vi "Máscaras registros.vi"(7 "Espera acceso USB:":u32, 8 "error in":errorcluster, 9 "Sumador-Salida":i32, 10 "Canal":i32, 11 "ftHandle_in":u32) -> (0 "error out":errorcluster, 1 "Scaler":i32, 2 "Num registro":i32, 3 "ftHandle_out":u32, 4 "DAC_MUX ENA":u16)   [LabVIEW 2009]
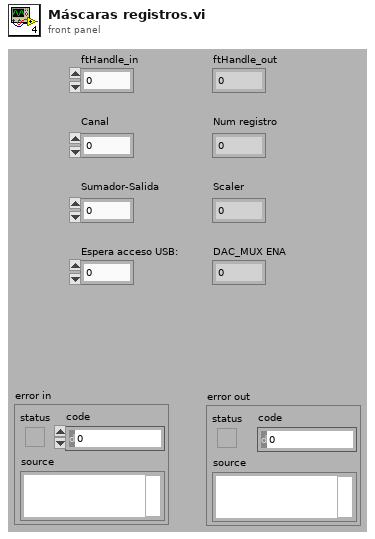
[diagram p1: front panel]
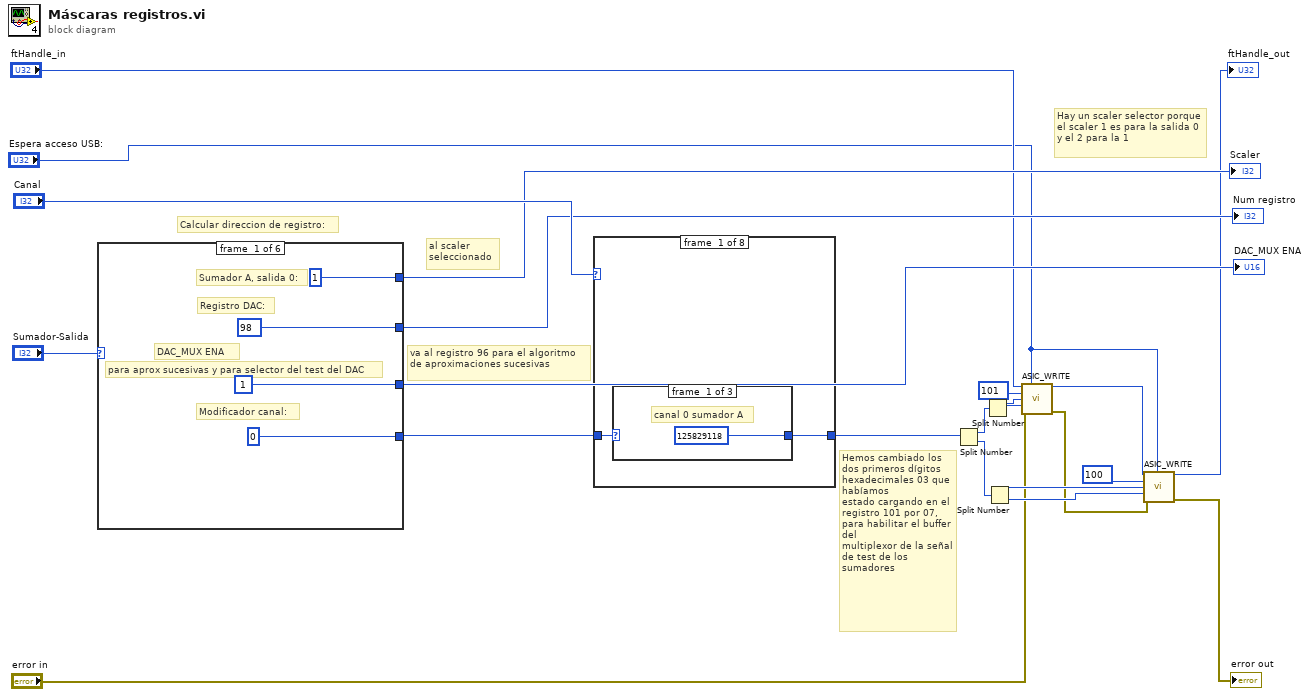
[diagram p0: block diagram]
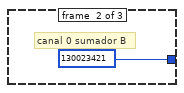
[diagram p2: hidden frame]
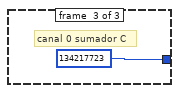
[diagram p3: hidden frame]
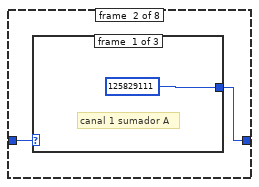
[diagram p4: hidden frame]
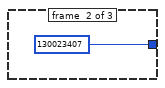
[diagram p5: hidden frame]
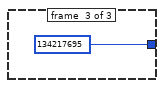
[diagram p6: hidden frame]
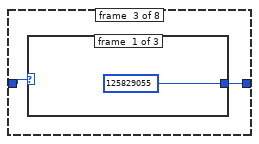
[diagram p7: hidden frame]
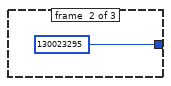
[diagram p8: hidden frame]
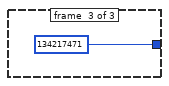
[diagram p9: hidden frame]
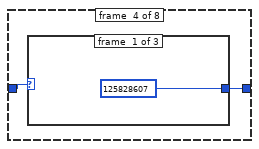
[diagram p10: hidden frame]
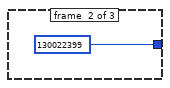
[diagram p11: hidden frame]
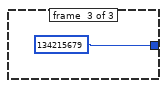
[diagram p12: hidden frame]
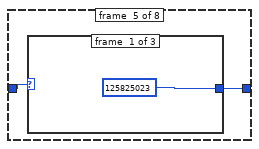
[diagram p13: hidden frame]
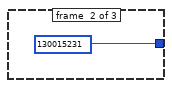
[diagram p14: hidden frame]
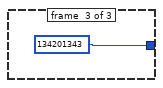
[diagram p15: hidden frame]
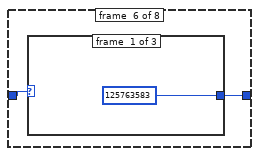
[diagram p16: hidden frame]
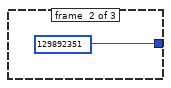
[diagram p17: hidden frame]
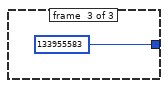
[diagram p18: hidden frame]
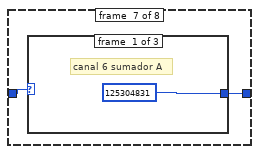
[diagram p19: hidden frame]
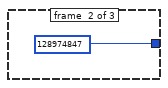
[diagram p20: hidden frame]
diagram:
  # "Hemos cambiado los dos primeros dígitos hexadecimales 03 que habíamos\nestado cargando en el registro 101 por 07, para habilitar el buffer del \nmultiplexor de la señal de test de los sumadores"
  # "Hay un scaler selector porque el scaler 1 es para la salida 0 y el 2 para la 1"
  # "al scaler\nseleccionado"
  # "va al registro 96 para el algoritmo de aproximaciones sucesivas"
  # "Calcular direccion de registro:"
  n1 = case shown="0, Default" "Sumador-Salida" {
    tunnel: [98 99 97 98 99 97] -> w12
    tunnel: [u16 1 2 3 4 5 6] -> w10
    tunnel: [0 1 2 0 1 2] -> w14
    tunnel: [1 1 1 2 2 2] -> w11
    frame #0 {
      # "para aprox sucesivas y para selector del test del DAC"
      # "Modificador canal:"
      # "DAC_MUX ENA"
      # "Registro DAC:"
      # "Sumador A, salida 0:"
    }
    frame #1 {
      # "Modificador canal:"
      # "Registro DAC:"
      # "Sumador B, salida 0:"
    }
    frame #2 {
      # "Modificador canal:"
      # "Registro DAC:"
      # "Sumador C, salida 0:"
    }
    frame #3 {
      # "Modificador canal:"
      # "Registro DAC:"
      # "Sumador A, salida 1:"
    }
    frame #4 {
      # "Modificador canal:"
      # "Registro DAC:"
      # "Sumador B, salida 1:"
    }
    frame #5 {
      # "Modificador canal:"
      # "Registro DAC:"
      # "Sumador C, salida 1:"
    }
  }
  "Num registro" <- w12
  "Scaler" <- w11
  "DAC_MUX ENA" <- w10
  n2 = case shown="1" "Canal" {
    tunnel: w14 -> [w48 w53 w58 w63 w68 w73 w78 w83]
    tunnel: [w47 w52 w57 w62 w67 w72 w77 w82] -> w1
    frame #0 {
      n3 = case shown="0, Default" w48 {
        tunnel: [u32 125829118 ("Threshold Inicial N") u32 130023421 ("Threshold Inicial N") u32 134217723 ("Threshold Inicial N")] -> w47
        frame #0 {
          # "canal 0 sumador A"
        }
        frame #1 {
          # "canal 0 sumador B"
        }
        frame #2 {
          # "canal 0 sumador C"
        }
      }
    }
    frame #1 {
      n4 = case shown="0, Default" w53 {
        tunnel: [u32 125829111 ("Threshold Inicial N") u32 130023407 ("Threshold Inicial N") u32 134217695 ("Threshold Inicial N")] -> w52
        frame #0 {
          # "canal 1 sumador A"
        }
        frame #1 {
        }
        frame #2 {
        }
      }
    }
    frame #2 {
      n5 = case shown="2" w58 {
        tunnel: [u32 125829055 ("Threshold Inicial N") u32 130023295 ("Threshold Inicial N") u32 134217471 ("Threshold Inicial N")] -> w57
        frame #0 {
        }
        frame #1 {
        }
        frame #2 {
        }
      }
    }
    frame #3 {
      n6 = case shown="2" w63 {
        tunnel: [u32 125828607 ("Threshold Inicial N") u32 130022399 ("Threshold Inicial N") u32 134215679 ("Threshold Inicial N")] -> w62
        frame #0 {
        }
        frame #1 {
        }
        frame #2 {
        }
      }
    }
    frame #4 {
      n7 = case shown="2" w68 {
        tunnel: [u32 125825023 ("Threshold Inicial N") u32 130015231 ("Threshold Inicial N") u32 134201343 ("Threshold Inicial N")] -> w67
        frame #0 {
        }
        frame #1 {
        }
        frame #2 {
        }
      }
    }
    frame #5 {
      n8 = case shown="2" w73 {
        tunnel: [u32 125763583 ("Threshold Inicial N") u32 129892351 ("Threshold Inicial N") u32 133955583 ("Threshold Inicial N")] -> w72
        frame #0 {
        }
        frame #1 {
        }
        frame #2 {
        }
      }
    }
    frame #6 {
      n9 = case shown="2" w78 {
        tunnel: [u32 125304831 ("Threshold Inicial N") u32 128974847 ("Threshold Inicial N") u32 132120575 ("Threshold Inicial N")] -> w77
        frame #0 {
          # "canal 6 sumador A"
        }
        frame #1 {
        }
        frame #2 {
        }
      }
    }
    frame #7 {
      # "caso especial para offset digital total\nde cada discriminador (todos los\ncanales abiertos a la vez)"
      n10 = case shown="0, Default" w83 {
        tunnel: [u32 125201846 ("Threshold Inicial N") u32 128801645 ("Threshold Inicial N") u32 131806939 ("Threshold Inicial N")] -> w82
        frame #0 {
          # "todos los canales sumador A"
        }
        frame #1 {
          # "todos los canales sumador B"
        }
        frame #2 {
          # "todos los canales sumador C"
        }
      }
    }
  }
  n11 = Split Number(x=w1) -> (hi(x)=w17:u16, lo(x)=w18:u16)
  n12 = Split Number(x=w17) -> (hi(x)=w19:u8, lo(x)=w20:u8)
  n13 = Split Number(x=w18) -> (hi(x)=w21:u8, lo(x)=w22:u8)
  n14 = call "ASIC_WRITE.vi"("ftHandle_in"="ftHandle_in", "Espera acceso USB"="Espera acceso USB:", "Direccion Registro Asic"=101, "Byte Alto"=w19, "Byte Bajo"=w20, "error in"="error in") -> ("ftHandle_out"=w7:u32, "error out"=w4:errorcluster)  [unwired: 8 in]
  n15 = call "ASIC_WRITE.vi"("ftHandle_in"=w7, "Espera acceso USB"="Espera acceso USB:", "Direccion Registro Asic"=100, "Byte Alto"=w21, "Byte Bajo"=w22, "error in"=w4) -> ("ftHandle_out"=→"ftHandle_out":u32, "error out"=→"error out":errorcluster)  [unwired: 8 in]
